vi "Stop Acquisition.vi"(8 "error in (no error)":errorcluster, 11 "Process in":refnum<class "Process.lvclass">) -> (0 "error out":errorcluster, 3 "Process out":refnum<class "Process.lvclass">)   [LabVIEW 2012, in "Process Actor.lvlib" / "Process.lvclass"]
doc: "This method will cause the actor to stop automatically sending data to the caller."
uses:
  Process.lvclass
  <vilib>/ActorFramework/Time-Delayed Send Message/Time-Delay Override Options.ctl
  Process.lvclass/Process.ctl
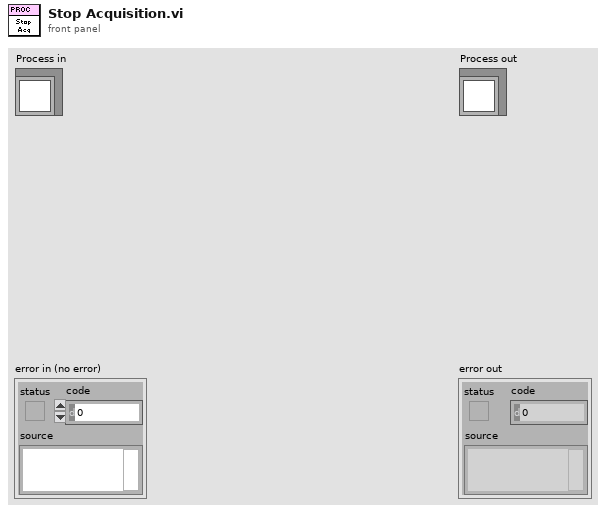
[diagram p1: front panel]
types:
  T1 = typedef "Time-Delay Override Options.ctl" = enum16{"Send next copy now", "Skip next scheduled copy", "Send next copy now and stop all further copies", "Stop all further copies"}
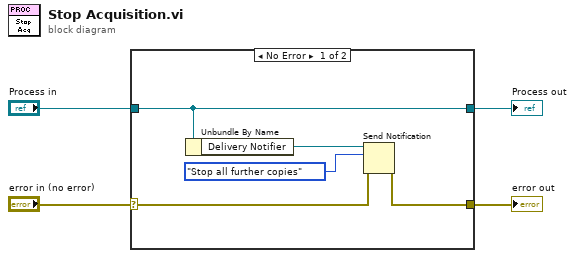
[diagram p0: block diagram]
diagram:
  n1 = case shown="No Error" "error in (no error)" {
    selector: "error in (no error)" -> [w6 w11]
    tunnel: [w5 w11] -> w3
    tunnel: [w9 w10] -> w1
    tunnel: "Process in" -> [w9 w10]
    frame No Error {
      n2 = Unbundle By Name(w9) -> ("Delivery Notifier"=w8:refnum<notifier>)
      n3 = Send Notification(notification=Time-Delay_Override_Options."Stop all further copies", notifier=w8, error in (no error)=w6) -> (error out=w5:errorcluster)  [unwired: 1 out]
    }
    frame Error {
    }
  }
  "error out" <- w3
  "Process out" <- w1
